vi "Choreo_DifferentialSample_Pack.vi"(9 "ChoreoDifferentialSample":T1={"timestamp"=-999.0, "x"=0.0, "y"=0.0, "heading"=0.0, "velocityL"=0.0, "velocityR"=0.0, "angularVelocity"=0.0, "accelL"=0.0, "accelR"=0.0, "accelAngular"=0.0, "forceL"=0.0, "forceR"=0.0}, 11 "RawData":u8[](array[numeric])) -> (3 "RawData Out":u8[](array[numeric]))   [LabVIEW 2019, in "ChoreoLib.lvlib"]
doc: "Pack a Differential Trajectory Sample cluster into a binary byte stream. New data will be added to the end of existing data.\n\nInputs:\n -- ChoreoDifferentialSample - cluster - Differential trajectory sample data\n -- RawData - Byte Array - Input byte stream\n \nOutputsL:\n -- RawData - Byte Array - Updated array of data."
uses:
  ChoreoLib.lvlib
  TypeDef/ChoreoDifferentialSample.ctl
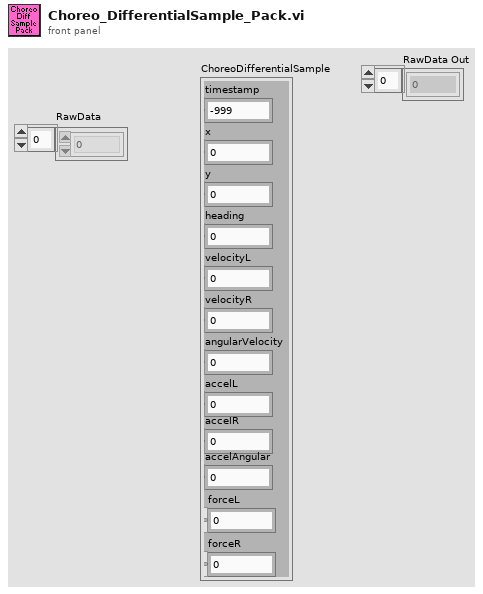
[diagram p1: front panel]
types:
  T1 = typedef "ChoreoLib.lvlib/ChoreoDifferentialSample.ctl" = cluster{"timestamp":dbl, "x":dbl, "y":dbl, "heading":dbl, "velocityL":dbl, "velocityR":dbl, "angularVelocity":dbl, "accelL":dbl, "accelR":dbl, "accelAngular":dbl, "forceL":dbl, "forceR":dbl}
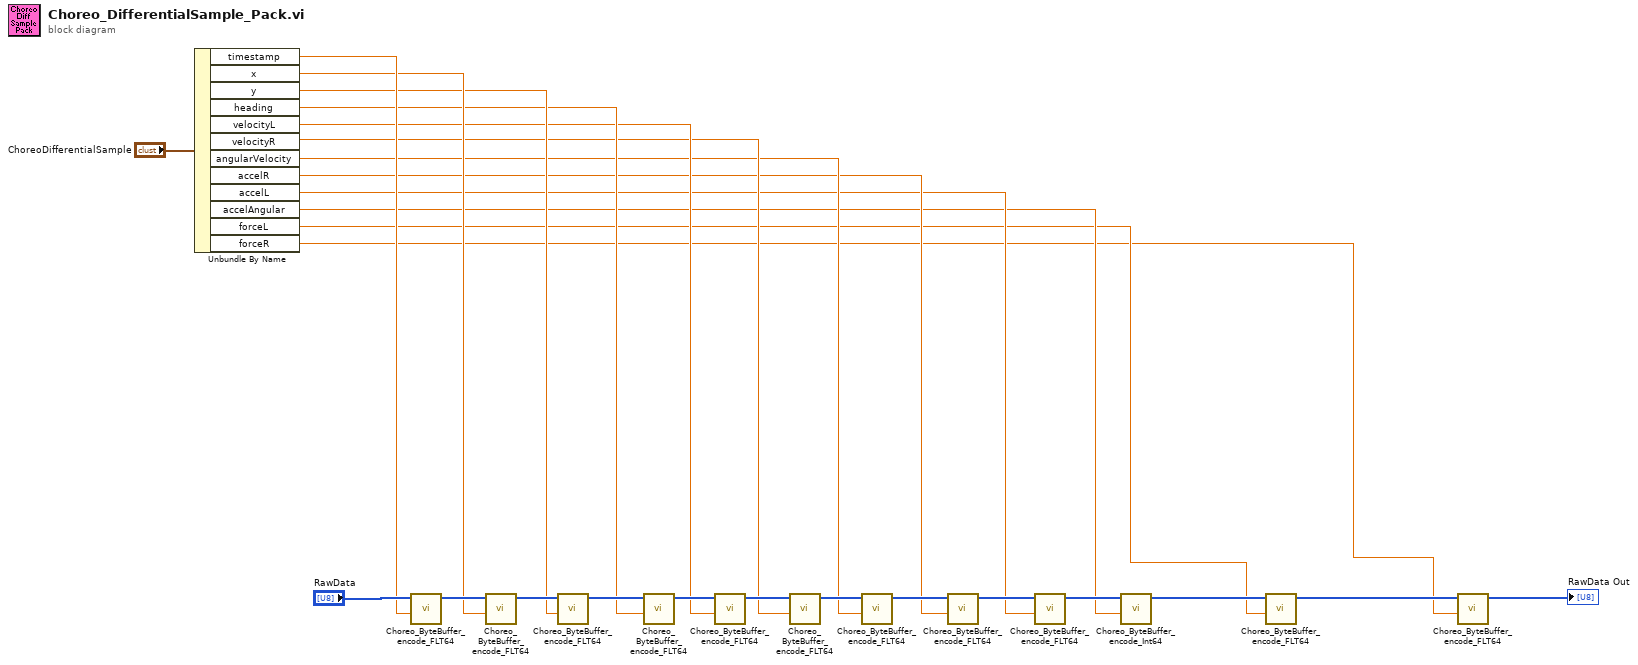
[diagram p0: block diagram]
diagram:
  n1 = Unbundle By Name("ChoreoDifferentialSample") -> ("timestamp"=w21:dbl, "x"=w20:dbl, "y"=w19:dbl, "heading"=w9:dbl, "velocityL"=w8:dbl, "velocityR"=w7:dbl, "angularVelocity"=w6:dbl, "accelR"=w5:dbl, "accelL"=w4:dbl, "accelAngular"=w3:dbl, "forceL"=w2:dbl, "forceR"=w1:dbl)
  n2 = call "Choreo_ByteBuffer_encode_FLT64.vi"("FLT64_Value"=w21, "RawData In"="RawData") -> ("RawData Out"=w23:u8[])  [unwired: 9 in]
  n3 = call "Choreo_ByteBuffer_encode_FLT64.vi"("FLT64_Value"=w20, "RawData In"=w23) -> ("RawData Out"=w22:u8[])  [unwired: 9 in]
  n4 = call "Choreo_ByteBuffer_encode_FLT64.vi"("FLT64_Value"=w19, "RawData In"=w22) -> ("RawData Out"=w18:u8[])  [unwired: 9 in]
  n5 = call "Choreo_ByteBuffer_encode_FLT64.vi"("FLT64_Value"=w9, "RawData In"=w18) -> ("RawData Out"=w17:u8[])  [unwired: 9 in]
  n6 = call "Choreo_ByteBuffer_encode_FLT64.vi"("FLT64_Value"=w8, "RawData In"=w17) -> ("RawData Out"=w16:u8[])  [unwired: 9 in]
  n7 = call "Choreo_ByteBuffer_encode_FLT64.vi"("FLT64_Value"=w7, "RawData In"=w16) -> ("RawData Out"=w15:u8[])  [unwired: 9 in]
  n8 = call "Choreo_ByteBuffer_encode_FLT64.vi"("FLT64_Value"=w6, "RawData In"=w15) -> ("RawData Out"=w14:u8[])  [unwired: 9 in]
  n9 = call "Choreo_ByteBuffer_encode_FLT64.vi"("FLT64_Value"=w5, "RawData In"=w14) -> ("RawData Out"=w13:u8[])  [unwired: 9 in]
  n10 = call "Choreo_ByteBuffer_encode_FLT64.vi"("FLT64_Value"=w4, "RawData In"=w13) -> ("RawData Out"=w12:u8[])  [unwired: 9 in]
  n11 = call "Choreo_ByteBuffer_encode_Int64.vi"("Int64_Value"=w3, "RawData In"=w12) -> ("RawData Out"=w11:u8[])  [unwired: 9 in]
  n12 = call "Choreo_ByteBuffer_encode_FLT64.vi"("FLT64_Value"=w2, "RawData In"=w11) -> ("RawData Out"=w25:u8[])  [unwired: 9 in]
  n13 = call "Choreo_ByteBuffer_encode_FLT64.vi"("FLT64_Value"=w1, "RawData In"=w25) -> ("RawData Out"=→"RawData Out":u8[])  [unwired: 9 in]
